vi "Close.vi"(7 "Stream":refnum<k24>, 8 "error in":errorcluster, 11 "SpreadsheetDoc":refnum<k24>) -> (0 "error out":errorcluster)   [LabVIEW 2019, in "Open Xml.lvlib"]
doc: "Not necessary when working with Editable = True on Open.vi"
uses:
  Open Xml.lvlib
  D:/git/Open-Xml-LabVIEW/Source/DocumentFormat.OpenXml.dll
  DocumentFormat.OpenXml.dll
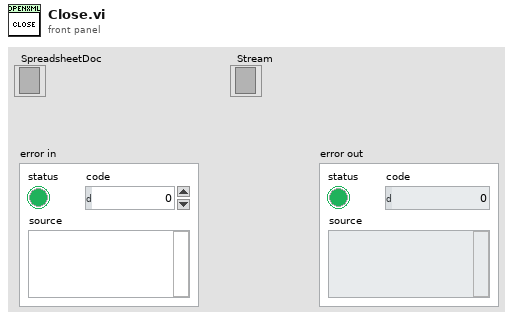
[diagram p1: front panel]
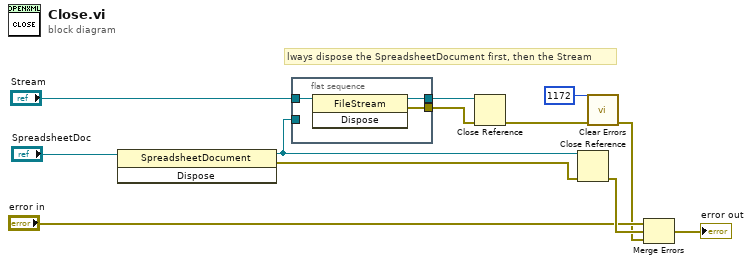
[diagram p0: block diagram]
diagram:
  # "lways dispose the SpreadsheetDocument first, then the Stream"
  n1 = invoke on="Invoke Node" class="SpreadsheetDocument" method="Dispose"(reference="SpreadsheetDoc") -> (reference out=w1:refnum<k24>, error out=w2:errorcluster)  [unwired: 2 in, 1 out]
  n2 = flat-sequence {
    tunnel: [w15] -> w9
    tunnel: "Stream" -> [w14]
    tunnel: [w13] -> w7
    tunnel: w1 -> [_]
    frame #0 {
      n3 = invoke class="FileStream" method="Dispose"(reference=w14) -> (reference out=w13:refnum<k24>, error out=w15:errorcluster)  [unwired: 2 in, 1 out]
    }
  }
  n4 = Close Reference(reference=w7, error in (no error)=w9) -> (error out=w6:errorcluster)
  n5 = Close Reference(reference=w1, error in (no error)=w2) -> (error out=w12:errorcluster)
  n6 = call <vilib>:"Clear Errors.vi"("error in (no error)"=w6, "specific error code to clear (0: all)"=1172) -> ("error out"=w4:errorcluster)  [unwired: 4 in, 1 out]
  n7 = Merge Errors("error in", w12, w4) -> (→"error out":errorcluster)
